vi "Update Build Version.vi"(8 "Error In":errorcluster, 11 "Target Project Root In":path) -> (0 "Error Out":errorcluster, 3 "Target Project Root Out":path)   [LabVIEW 2017]
doc: "Copies the build specification from the target previous version, where the build version has been autoincremented, to the VIPB for the trunk/source project."
uses:
  <vilib>/JKI/VIPM API/VIPM API_vipm_api.lvlib
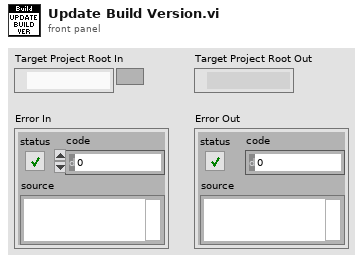
[diagram p1: front panel]
types:
  T1 = typedef "VIPM API_vipm_api.lvlib/VI Package Build Spec Data Cluster_vipm_api.ctl" = cluster{"Package Version":T2, "Product Name":string, "Company Name":string, "Author Name (Person or Company)":string, "Product Homepage (URL)":string, "Legal Copyright":string, "License Agreement Name":string, "Product Description Summary":string, "Product Description":string, "Release Notes - Change Log":string}
  T2 = typedef "VIPM API_vipm_api.lvlib/Version Info Cluster_vipm_api.ctl" = cluster{"major":u32, "minor":u32, "patch":u32, "build":u32}
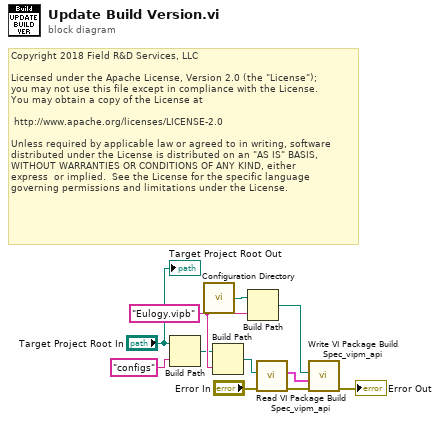
[diagram p0: block diagram]
diagram:
  w10 = "Eulogy.vipb" ("name or relative path")
  # "Copyright 2018 Field R&D Services, LLC\n\nLicensed under the Apache License, Version 2.0 (the \"License\");\nyou may not use this file except in compliance with the License.\nYou may obtain a copy of the License at\n\n\thttp://www.apache.org/licenses/LICENSE-2.0\n\nUnless required by applicable law or agreed to in writing, software\ndistributed under the License is distributed on an \"AS IS\" BASIS,\nWITHOUT WARRANTIES OR CONDITIONS OF ANY KIND, either \nexpress  or implied.  See the License for the specific language \ngoverning permissions and limitations under the License."
  n1 = Build Path(base path="Target Project Root In", name or relative path="configs") -> (appended path=w3:path)
  n2 = call "Configuration Directory.vi"() -> ("Configuration Directory"=w9:path)
  n3 = Build Path(base path=w3, name or relative path=w10) -> (appended path=w4:path)
  n4 = Build Path(base path=w9, name or relative path=w10) -> (appended path=w11:path)
  n5 = call <vilib>:"Read VI Package Build Spec_vipm_api.vi"("error in (no error)"="Error In", "Path to VIPB File"=w4) -> ("error out"=w7:errorcluster, "VI Package Build Spec Data"=w6:T1)  [unwired: 8 in]
  n6 = call <vilib>:"Write VI Package Build Spec_vipm_api.vi"("error in (no error)"=w7, "VI Package Build Spec Data"=w6, "Path to VIPB File"=w11) -> ("error out"=→"Error Out":errorcluster)  [unwired: 8 in]
  "Target Project Root Out" <- "Target Project Root In"
